vi "3654DriveStraight.vi"(11 "X-AxisIn":dbl) -> (3 "X-AxisOut":dbl)   [LabVIEW 2017]
uses:
  Robot Global Data.vi
  <vilib>/Rock Robotics/WPI/ThirdParty/Phoenix-LabVIEW/Pigeon IMU/CTRE_PigeonIMU_GetFusedHeading.vi
  <vilib>/addons/control/pid/pid.llb/PID (DBL).vi
  <vilib>/addons/control/pid/NI_PID_pid.lvlib
panel:
  out "Heading":dbl
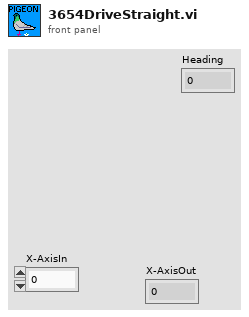
[diagram p1: front panel]
types:
  T1 = typedef "CTRE_PigeonIMU_DeviceRef.ctl" = cluster{"DeviceStatus":errorcluster, "Device Number":u8, "Type":T2, "Device ID":u32, "Handle":u64, "UsageFrame":u32, "Library Path":path}
  T2 = typedef "CTRE_PigeonIMU_ConnectionType.ctl" = u32
  T3 = cluster{"Heading":dbl, "Valid?":bool, "Fusing?":bool}
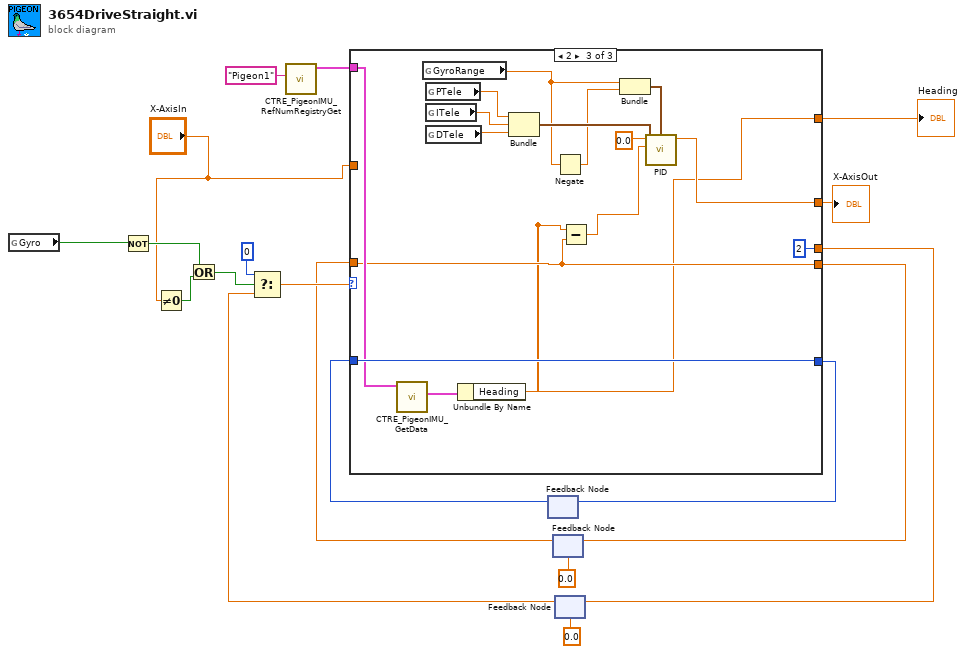
[diagram p0: block diagram]
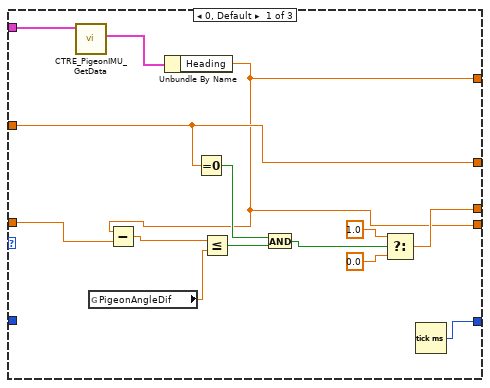
[diagram p2: hidden frame]
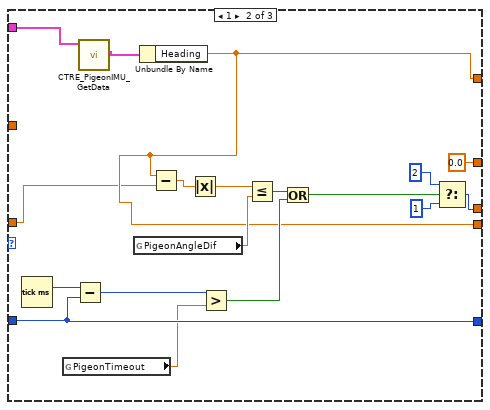
[diagram p3: hidden frame]
diagram:
  n1 = global read "Robot Global Data.vi" "Gyro"() -> (w7:bool)
  n2 = Not(x=w7) -> (.not. x?=w19:bool)
  n3 = Not Equal To 0?(x="X-AxisIn") -> (x != 0?=w18:bool)
  n4 = Or(x=w19, y=w18) -> (x .or. y?=w17:bool)
  n5 = call <vilib>:"CTRE_PigeonIMU_RefNumRegistryGet.vi"("refnum name"="Pigeon1") -> ("PigeonIMUDevRef"=w5:T1)  [unwired: 9 in, 1 out]
  n6 = feedback #1() -> (w10:u32)  [unwired: 1 in]
  n7 = feedback #2(0.0 ("Yaw")) -> (w8:dbl)
  n8 = feedback #3(0.0 ("f")) -> (w12:dbl)
  n9 = Select(t=0, s=w17, f=w12) -> (s? t:f=w16:dbl)
  n10 = case shown="2" w16 {
    tunnel: "X-AxisIn" -> [w25 _ _]
    tunnel: [w25 0.0 ("X-AxisIn") w57] -> w14
    tunnel: [w30 w42 2] -> w13
    tunnel: [w33 w47 w66] -> w11
    tunnel: w10 -> [_ w47 w66]
    tunnel: [w21 w35 w54] -> w3
    tunnel: w8 -> [w20 w34 w54]
    tunnel: w5 -> [w32 w40 w56]
    tunnel: [w21 w35 w53] -> w2
    frame 0, Default {
      n11 = call-poly <vilib>:"CTRE_PigeonIMU_GetData.vi"("PigeonIMUDevRef"=w32) -> ("Fused Heading"=w31:T3)  [unwired: 8 in, 2 out]
      n12 = global read "Robot Global Data.vi" "PigeonAngleDif"() -> (w29:dbl)
      n13 = Unbundle By Name(w31) -> ("Heading"=w21:dbl)
      n14 = Subtract(x=w21, y=w20) -> (x-y=w22:dbl)
      n15 = Equal To 0?(x=w25) -> (x = 0?=w24:bool)
      n16 = Less Or Equal?(x=w22, y=w29) -> (x <= y?=w26:bool)
      n17 = And(x=w24, y=w26) -> (x .and. y?=w23:bool)
      n18 = Select(t=1.0, s=w23, f=0.0) -> (s? t:f=w30:dbl)
      n19 = Tick Count (ms)() -> (millisecond timer value=w33:u32)
    }
    frame 1 {
      n20 = Tick Count (ms)() -> (millisecond timer value=w49:u32)
      n21 = global read "Robot Global Data.vi" "PigeonTimeout"() -> (w37:dbl)
      n22 = Subtract(x=w49, y=w47) -> (x-y=w48:u32)
      n23 = call-poly <vilib>:"CTRE_PigeonIMU_GetData.vi"("PigeonIMUDevRef"=w40) -> ("Fused Heading"=w39:T3)  [unwired: 8 in, 2 out]
      n24 = global read "Robot Global Data.vi" "PigeonAngleDif"() -> (w38:dbl)
      n25 = Unbundle By Name(w39) -> ("Heading"=w35:dbl)
      n26 = Subtract(x=w35, y=w34) -> (x-y=w36:dbl)
      n27 = Absolute Value(x=w36) -> (abs(x)=w51:dbl)
      n28 = Greater?(x=w48, y=w37) -> (0:w46:bool)
      n29 = Less Or Equal?(x=w51, y=w38) -> (x <= y?=w50:bool)
      n30 = Or(x=w50, y=w46) -> (x .or. y?=w45:bool)
      n31 = Select(t=2, s=w45, f=1) -> (s? t:f=w42:i32)
    }
    frame 2 {
      n32 = call-poly <vilib>:"CTRE_PigeonIMU_GetData.vi"("PigeonIMUDevRef"=w56) -> ("Fused Heading"=w55:T3)  [unwired: 8 in, 2 out]
      n33 = global read "Robot Global Data.vi" "GyroRange"() -> (w58:dbl)
      n34 = global read "Robot Global Data.vi" "PTele"() -> (w65:dbl)
      n35 = global read "Robot Global Data.vi" "ITele"() -> (w64:dbl)
      n36 = global read "Robot Global Data.vi" "DTele"() -> (w63:dbl)
      n37 = Unbundle By Name(w55) -> ("Heading"=w53:dbl)
      n38 = Bundle("PTele"=w65, "ITele"=w64, "DTele"=w63) -> (w62:cluster{"PTele":dbl, "ITele":dbl, "DTele":dbl})  [unwired: 1 in]
      n39 = Negate(x=w58) -> (-x=w59:dbl)
      n40 = Subtract(x=w53, y=w54) -> (x-y=w52:dbl)
      n41 = Bundle("GyroRange"=w58, w59) -> (w60:cluster{"GyroRange":dbl, dbl})  [unwired: 1 in]
      n42 = call-poly <vilib>:"PID.vi"("output range"=w60, "PID gains"=w62, "process variable"=w52, "setpoint"=0.0) -> ("output"=w57:dbl)  [unwired: 6 in, 1 out]
    }
  }
  "X-AxisOut" <- w14
  "Heading" <- w2
  n43 = feedback-in #1(w11) -> ()
  n44 = feedback-in #2(w3) -> ()
  n45 = feedback-in #3(w13) -> ()
